vi "SwerveChooseAngle_Luke.vi"(2 "Hysteresis (deg)":dbl=10.0 format="%#_13g", 3 "Goal Angle (deg)":dbl format="%#_13g", 4 "Current Angle (deg)":dbl format="%#_13g") -> (0 "Invert Speed  Motor (?)":bool, 1 "Angular Distance (deg)":dbl format="%_4g")   [LabVIEW 2018]
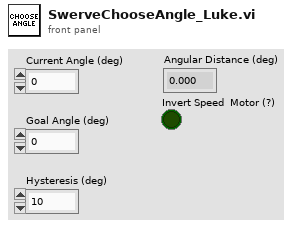
[diagram p1: front panel]
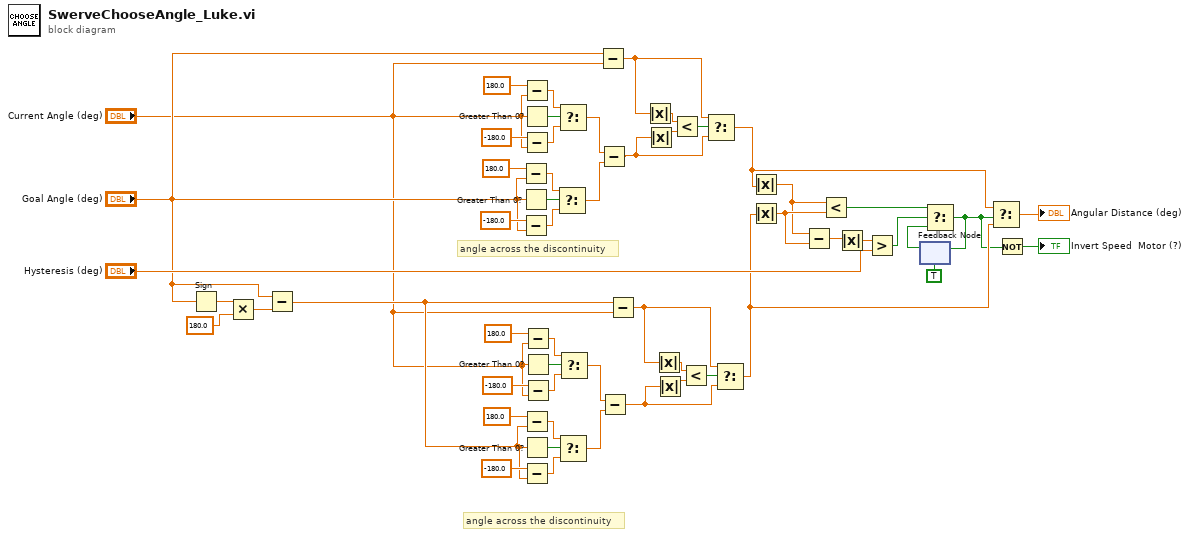
[diagram p0: block diagram]
diagram:
  # "angle across the discontinuity"
  # "angle across the discontinuity"
  n1 = Sign(1:"Goal Angle (deg)") -> (0:w54:dbl)
  n2 = Multiply(x=w54, y=180.0) -> (x*y=w52:dbl)
  n3 = Subtract(x="Goal Angle (deg)", y=w52) -> (x-y=w22:dbl)
  n4 = Subtract(x=180.0, y="Goal Angle (deg)") -> (x-y=w9:dbl)
  n5 = Greater Than 0?(x="Goal Angle (deg)") -> (x > 0?=w11:bool)
  n6 = Subtract(x=-180.0, y="Goal Angle (deg)") -> (x-y=w7:dbl)
  n7 = Subtract(x=180.0, y="Current Angle (deg)") -> (x-y=w14:dbl)
  n8 = Greater Than 0?(x="Current Angle (deg)") -> (x > 0?=w16:bool)
  n9 = Subtract(x=-180.0, y="Current Angle (deg)") -> (x-y=w12:dbl)
  n10 = Subtract(x=180.0, y=w22) -> (x-y=w31:dbl)
  n11 = Greater Than 0?(x=w22) -> (x > 0?=w33:bool)
  n12 = Subtract(x=-180.0, y=w22) -> (x-y=w29:dbl)
  n13 = Subtract(x=180.0, y="Current Angle (deg)") -> (x-y=w38:dbl)
  n14 = Greater Than 0?(x="Current Angle (deg)") -> (x > 0?=w40:bool)
  n15 = Subtract(x=-180.0, y="Current Angle (deg)") -> (x-y=w36:dbl)
  n16 = Select(t=w9, s=w11, f=w7) -> (s? t:f=w5:dbl)
  n17 = Select(t=w14, s=w16, f=w12) -> (s? t:f=w6:dbl)
  n18 = Select(t=w31, s=w33, f=w29) -> (s? t:f=w27:dbl)
  n19 = Select(t=w38, s=w40, f=w36) -> (s? t:f=w28:dbl)
  n20 = Subtract(x="Goal Angle (deg)", y="Current Angle (deg)") -> (x-y=w17:dbl)
  n21 = Subtract(x=w6, y=w5) -> (x-y=w2:dbl)
  n22 = Subtract(x=w28, y=w27) -> (x-y=w26:dbl)
  n23 = Subtract(x=w22, y="Current Angle (deg)") -> (x-y=w23:dbl)
  n24 = Absolute Value(x=w17) -> (abs(x)=w19:dbl)
  n25 = Absolute Value(x=w2) -> (abs(x)=w20:dbl)
  n26 = Absolute Value(x=w23) -> (abs(x)=w24:dbl)
  n27 = Absolute Value(x=w26) -> (abs(x)=w25:dbl)
  n28 = Less?(x=w19, y=w20) -> (x < y?=w21:bool)
  n29 = Less?(x=w24, y=w25) -> (x < y?=w35:bool)
  n30 = Select(t=w17, s=w21, f=w2) -> (s? t:f=w18:dbl)
  n31 = Select(t=w23, s=w35, f=w26) -> (s? t:f=w34:dbl)
  n32 = Absolute Value(x=w18) -> (abs(x)=w42:dbl)
  n33 = Absolute Value(x=w34) -> (abs(x)=w43:dbl)
  n34 = Subtract(x=w42, y=w43) -> (x-y=w47:dbl)
  n35 = Less?(x=w42, y=w43) -> (x < y?=w41:bool)
  n36 = Absolute Value(x=w47) -> (abs(x)=w46:dbl)
  n37 = Greater?(x=w46, y="Hysteresis (deg)") -> (0:w44:bool)
  n38 = feedback #1(TRUE) -> (w49:bool)
  n39 = Select(t=w41, s=w44, f=w49) -> (s? t:f=w1:bool)
  n40 = feedback-in #1(w1) -> ()
  n41 = Select(t=w18, s=w1, f=w34) -> (s? t:f=→"Angular Distance (deg)":dbl)
  n42 = Not(x=w1) -> (.not. x?=→"Invert Speed  Motor (?)":bool)
